vi "Launch Topic.vi"(7 "Include Initial Value? (F)":bool, 9 "Type":variant, 10 "Datum Name":string, 11 "MonitoredMediator in":refnum<class "MonitoredMediator.lvclass">) -> (0 "error out":errorcluster, 2 "New Topic Enqueuer":refnum<class "Message Enqueuer.lvclass">, 3 "MonitoredMediator out":refnum<class "MonitoredMediator.lvclass">)   [LabVIEW 2018, in "MVA Framework.lvlib" / "MonitoredMediator.lvlib" / "MonitoredMediator.lvclass"]
uses:
  MonitoredMediator.lvclass
  Mediator/Topic Messages/Add Topic Subscriber Msg/Add Topic Subscriber Msg.lvclass
  IMediator/ISubscriptionPolicy/ISubscriptionPolicy.lvclass
  IBusMonitor/IBusMonitor.lvclass
  Mediator/Mediator/Mediator.lvclass
  <vilib>/ActorFramework/Message Enqueuer/Message Enqueuer.lvclass
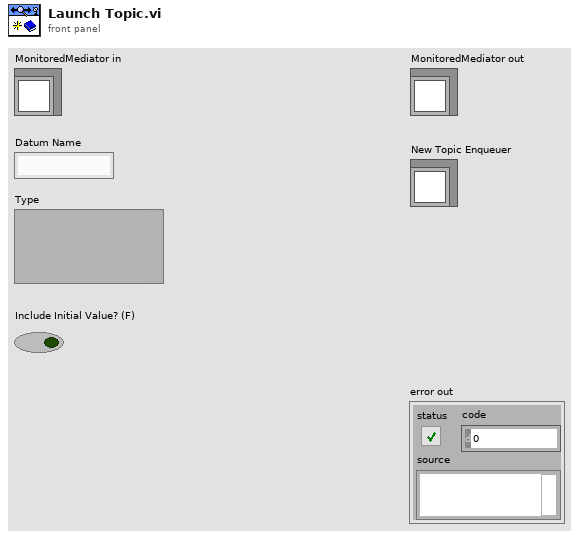
[diagram p1: front panel]
types:
  T1 = typedef "MVA Framework.lvlib/IMediator.lvlib/ISubscriptionPolicy.lvclass/ISubscriptionPolicy Reference.ctl" = refnum<data-value>
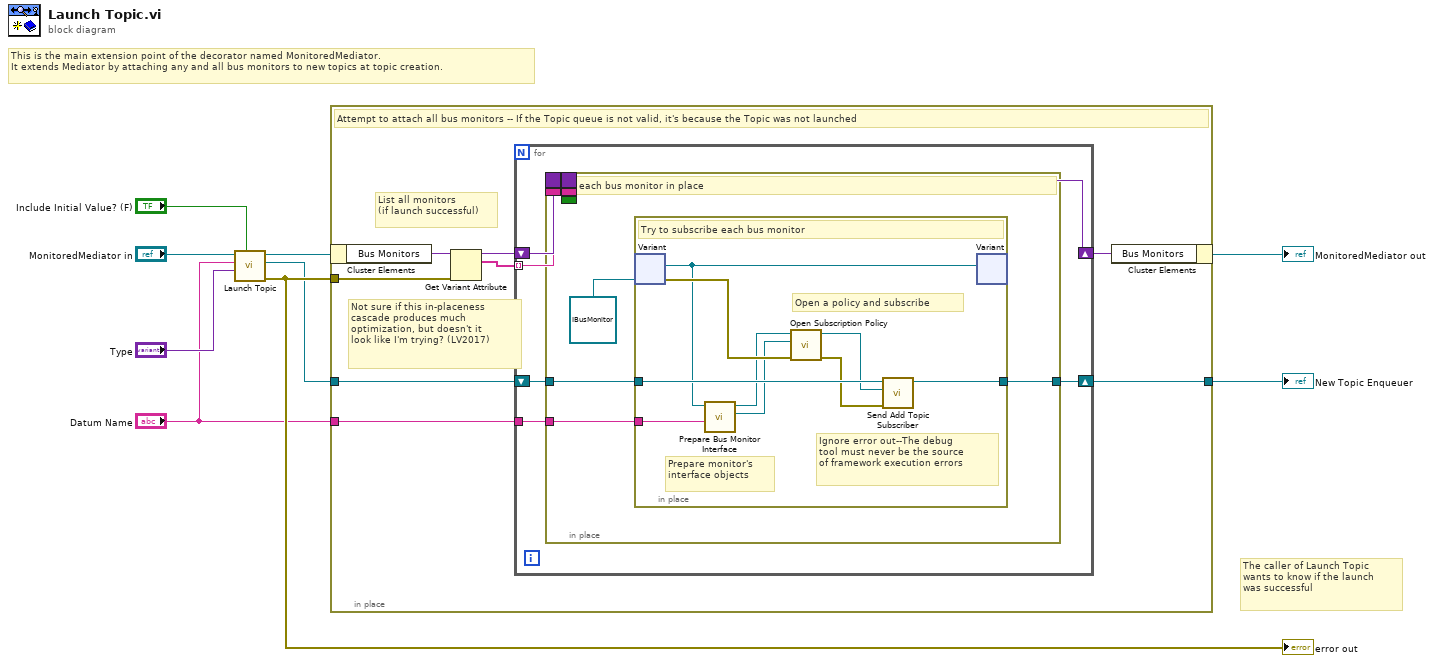
[diagram p0: block diagram]
diagram:
  # "The caller of Launch Topic\nwants to know if the launch\nwas successful"
  # "This is the main extension point of the decorator named MonitoredMediator.\nIt extends Mediator by attaching any and all bus monitors to new topics at topic creation."
  n1 = call-parent "Launch Topic.vi"("Include Initial Value? (F)"="Include Initial Value? (F)", "Type"="Type", "Datum Name"="Datum Name", "Mediator in"="MonitoredMediator in") -> ("error out"=w3:errorcluster, "New Topic Enqueuer"=w2:refnum<class "Message Enqueuer.lvclass">, "Mediator out"=w4:refnum<class "MonitoredMediator.lvclass">)  [unwired: 5 in]
  "error out" <- w3
  n2 = in-place {
    in-place-border: w2 -> [w17]
    in-place-border: [w16] -> w7
    in-place-border: w3 -> [w11]
    in-place-border: "Datum Name" -> [w10]
    # "Not sure if this in-placeness\ncascade produces much\noptimization, but doesn't it\nlook like I'm trying? (LV2017)"
    # "List all monitors\n(if launch successful)"
    # "Attempt to attach all bus monitors -- If the Topic queue is not valid, it's because the Topic was not launched"
    n3 = in-place-cluster #1(w4) -> ("Bus Monitors"=w14:variant)
    n4 = Get Variant Attribute(Variant=w14, error in=w11) -> (duplicate Variant=w13:variant, names=w12:string[])  [unwired: 2 in, 2 out]
    n5 = for {
      shift-right: [w22] -> w16
      shift-left: w17 -> [w23]
      tunnel: w12 -> [w19] mode=indexing
      tunnel: w10 -> [w18]
      shift-right: [w21] -> w15
      shift-left: w13 -> [w20]
      n6 = in-place {
        in-place-border: w23 -> [w29]
        in-place-border: [w28] -> w22
        border: w20 -> [_]
        border: w19 -> [_]
        border: [_] -> w21
        border: _ -> [_]
        border: _ -> [_]
        in-place-border: w18 -> [w24]
        # "Read each bus monitor in place"
        n7 = in-place {
          in-place-border: w29 -> [w38]
          in-place-border: [w36] -> w28
          in-place-border: w24 -> [w31]
          # "Ignore error out--The debug\ntool must never be the source\nof framework execution errors"
          # "Open a policy and subscribe"
          # "Prepare monitor's\ninterface objects"
          # "Try to subscribe each bus monitor"
          n8 = in-place-variant #2(w27, refnum<class "IBusMonitor.lvclass"> refnum ("IBusMonitor")) -> (w30:refnum<class "IBusMonitor.lvclass">, w34:errorcluster)
          n9 = call-dynamic "Prepare Bus Monitor Interface.vi"("Datum Name"=w31, "IBusMonitor"=w30) -> ("Valid Transport"=w32:refnum<class "ITransport.lvclass">, "SubscriptionPolicy"=w33:refnum<class "ISubscriptionPolicy.lvclass">)  [unwired: 8 in]
          n10 = call "Open Subscription Policy.vi"("error in (no error)"=w34, "Transport"=w32, "SubscriptionPolicy"=w33) -> ("error out"=w35:errorcluster, "Subscription Policy"=w37:T1)  [unwired: 7 in]
          n11 = call "Send Add Topic Subscriber.vi"("error in (no error)"=w35, "Subscription Policy"=w37, "Message Enqueuer"=w38) -> ("Message Enqueuer out"=w36:refnum<class "Message Enqueuer.lvclass">)  [unwired: 7 in, 1 out]
          n12 = in-place-variant #2(w30) -> (w26:variant)  [unwired: 1 out]
        }
      }
    }
    n13 = in-place-cluster #1("Bus Monitors"=w15) -> (→"MonitoredMediator out":refnum<class "MonitoredMediator.lvclass">)
  }
  "New Topic Enqueuer" <- w7
